vi "Measurer.vi"() -> ()   [LabVIEW 2019]
uses:
  <vilib>/Analysis/baseanly.llb/Mean (DBL).vi
  Components/DeltaRamp_globals.vi
  Components/B_Globals.vi
  Components/Global 2.vi
  Components/ReadLockGlobals.vi
  <vilib>/Analysis/NI_AALBase.lvlib
panel:
  out "T_Set [K]":dbl=1.5
  out "R4":cluster{"X":dbl[], "Y":dbl[]}[](graph)=[{"X"=[1.7047999999999999, 1.7049, 1.7048000000000003, 1.7049, 1.7048000000000003, 1.7049, 1.705, 1.7049, 1.705, 1.7048000000000003, 1.7047000000000003, 1.7045999999999997, 1.7047000000000012, 1.7047999999999999, 1.7045999999999994, 1.7044999999999997, 1.7045999999999997, 1.7044999999999997, 1.7045999999999994, 1.7044999999999997, 1.7046, 1.7044999999999997, 1.7044, 1.7044999999999997, 1.7044, 1.7043, 1.7044, 1.7044999999999997, 1.7044000000000001, 1.7044999999999997, 1.7047000000000003, 1.7045999999999997, 1.7044999999999997, 1.7045999999999997, 1.7046999999999999, 1.7045999999999997, 1.7046999999999999, 1.7048000000000003, 1.7047000000000003, 1.7047999999999994, 1.7049, 1.7047999999999999, 1.7047, 1.7048000000000003, 1.7045999999999997, 1.7047, 1.7048000000000003, 1.7049, 1.7048000000000003], "Y"=[]}] caption="XY Graph"
  out "R [Ohm]":dbl[](array[numeric])=[0.218917653]
  out "Array":T1(array[cluster])=[{"Name"="AEN056B", "Measurment Type"="6221 - Delta", "I Max"=1e-05, "Freq/Delay"=0.002, "Address"="GPIB1::20::INSTR", "Enabled"=FALSE}, {"Name"="CrossJunction_device5", "Measurment Type"="6221 - Delta", "I Max"=1e-05, "Freq/Delay"=0.002, "Address"="GPIB1::22::INSTR", "Enabled"=TRUE}]
  in  "Config":bool
  in  "Graphing":string(combo)="Single"
  out "T 3":cluster{"X":dbl[], "Y":dbl[]}[](graph)=[{"X"=[1.7047999999999999, 1.7049, 1.7048000000000003, 1.7049, 1.7048000000000003, 1.7049, 1.705, 1.7049, 1.705, 1.7048000000000003, 1.7047000000000003, 1.7045999999999997, 1.7047000000000012, 1.7047999999999999, 1.7045999999999994, 1.7044999999999997, 1.7045999999999997, 1.7044999999999997, 1.7045999999999994, 1.7044999999999997, 1.7046, 1.7044999999999997, 1.7044, 1.7044999999999997, 1.7044, 1.7043, 1.7044, 1.7044999999999997, 1.7044000000000001, 1.7044999999999997, 1.7047000000000003, 1.7045999999999997, 1.7044999999999997, 1.7045999999999997, 1.7046999999999999, 1.7045999999999997, 1.7046999999999999, 1.7048000000000003, 1.7047000000000003, 1.7047999999999994, 1.7049, 1.7047999999999999, 1.7047, 1.7048000000000003, 1.7045999999999997, 1.7047, 1.7048000000000003, 1.7049, 1.7048000000000003], "Y"=[]}] caption="XY Graph"
  out "T 2":cluster{"X":dbl[], "Y":dbl[]}[](graph)=[{"X"=[1.7047999999999999, 1.7049, 1.7048000000000003, 1.7049, 1.7048000000000003, 1.7049, 1.705, 1.7049, 1.705, 1.7048000000000003, 1.7047000000000003, 1.7045999999999997, 1.7047000000000012, 1.7047999999999999, 1.7045999999999994, 1.7044999999999997, 1.7045999999999997, 1.7044999999999997, 1.7045999999999994, 1.7044999999999997, 1.7046, 1.7044999999999997, 1.7044, 1.7044999999999997, 1.7044, 1.7043, 1.7044, 1.7044999999999997, 1.7044000000000001, 1.7044999999999997, 1.7047000000000003, 1.7045999999999997, 1.7044999999999997, 1.7045999999999997, 1.7046999999999999, 1.7045999999999997, 1.7046999999999999, 1.7048000000000003, 1.7047000000000003, 1.7047999999999994, 1.7049, 1.7047999999999999, 1.7047, 1.7048000000000003, 1.7045999999999997, 1.7047, 1.7048000000000003, 1.7049, 1.7048000000000003], "Y"=[0.19752289130769227, 0.20950811671428574, 0.1808979382857143, 0.17235231225, 0.17432194683333332, 0.2235183616666667, 0.21412651671428576, 0.20596404375999997, 0.2051939327142857, 0.20028577114285714, 0.19771953790909091, 0.20788647657142859, 0.19616624683333334, 0.1948073679230769, 0.2037684524285714, 0.196056151, 0.196453916, 0.19739343871428575, 0.21256366375, 0.1747552657, 0.15625726666666667, 0.19934746358333333, 0.19194195983333331, 0.19936784685714287, 0.2009971615357143, 0.21071373433333332, 0.20681018633333334, 0.20449920628571427, 0.1755347936, 0.20595055476923077, 0.20658881114285715, 0.21645730942857141, 0.20386924071428572, 0.1994578533809524, 0.20553432800000002, 0.21412651242857142, 0.20646832086666667, 0.2077425187142857, 0.218575714, 0.20290053768181818, 0.17640915285714284, 0.19304051792857146, 0.209842004, 0.2081186685714286, 0.20430601066666668, 0.20083773000000002, 0.19869472714285713, 0.20326516587499996, 0.20483756485714283]}] caption="XY Graph"
  in  "Clear Paths":bool
  out "Remote Inherit Path":path=path "C:/User Data/gy251/20210406 EuS10-Cu (t)-EuS20/Delta_500uA_RH_T=16p00K.txt"
  in  "Remote Directory":path=path "C:/User Data/gy251/20210811 Cross junction for Oded/Device 5_750 nm width/Junction check_7-8-10-11"
  out "Last Saved":path=path "C:/User Data/gy251/20210810 AEN056B/JJ8/CrossJunction_device5_RT_10uA_cool.txt"
  in  "Remote_Save_String [This is the important one!]":string="RT_10uA_warm"
  out "B_set [T]":dbl
  in  "Reading Delay [ms]":i32=20 min=5
  in  "RW Delay":i32=10
  out "Exec Time [ms]":u32=39
  in  "B/T":bool=TRUE
  in  "Smart Avs":bool=TRUE
  in  "Points":dbl=1.0
  out "PpP":dbl=7.0
  in  "Combo Box":string(combo)="Temp"
  in  "Save":bool
  in  "Abort":bool
  out "B [T]":dbl
  in  "Arm":bool
  in  "Measure":bool
  out "T":cluster{"X":dbl[], "Y":dbl[]}[](graph)=[{"X"=[1.7047999999999999, 1.7049, 1.7048000000000003, 1.7049, 1.7048000000000003, 1.7049, 1.705, 1.7049, 1.705, 1.7048000000000003, 1.7047000000000003, 1.7045999999999997, 1.7047000000000012, 1.7047999999999999, 1.7045999999999994, 1.7044999999999997, 1.7045999999999997, 1.7044999999999997, 1.7045999999999994, 1.7044999999999997, 1.7046, 1.7044999999999997, 1.7044, 1.7044999999999997, 1.7044, 1.7043, 1.7044, 1.7044999999999997, 1.7044000000000001, 1.7044999999999997, 1.7047000000000003, 1.7045999999999997, 1.7044999999999997, 1.7045999999999997, 1.7046999999999999, 1.7045999999999997, 1.7046999999999999, 1.7048000000000003, 1.7047000000000003, 1.7047999999999994, 1.7049, 1.7047999999999999, 1.7047, 1.7048000000000003, 1.7045999999999997, 1.7047, 1.7048000000000003, 1.7049, 1.7048000000000003], "Y"=[0.19752289130769227, 0.20950811671428574, 0.1808979382857143, 0.17235231225, 0.17432194683333332, 0.2235183616666667, 0.21412651671428576, 0.20596404375999997, 0.2051939327142857, 0.20028577114285714, 0.19771953790909091, 0.20788647657142859, 0.19616624683333334, 0.1948073679230769, 0.2037684524285714, 0.196056151, 0.196453916, 0.19739343871428575, 0.21256366375, 0.1747552657, 0.15625726666666667, 0.19934746358333333, 0.19194195983333331, 0.19936784685714287, 0.2009971615357143, 0.21071373433333332, 0.20681018633333334, 0.20449920628571427, 0.1755347936, 0.20595055476923077, 0.20658881114285715, 0.21645730942857141, 0.20386924071428572, 0.1994578533809524, 0.20553432800000002, 0.21412651242857142, 0.20646832086666667, 0.2077425187142857, 0.218575714, 0.20290053768181818, 0.17640915285714284, 0.19304051792857146, 0.209842004, 0.2081186685714286, 0.20430601066666668, 0.20083773000000002, 0.19869472714285713, 0.20326516587499996, 0.20483756485714283]}] caption="XY Graph"
  in  "Reset":bool
  out "Spl T [K]":dbl=1.7047
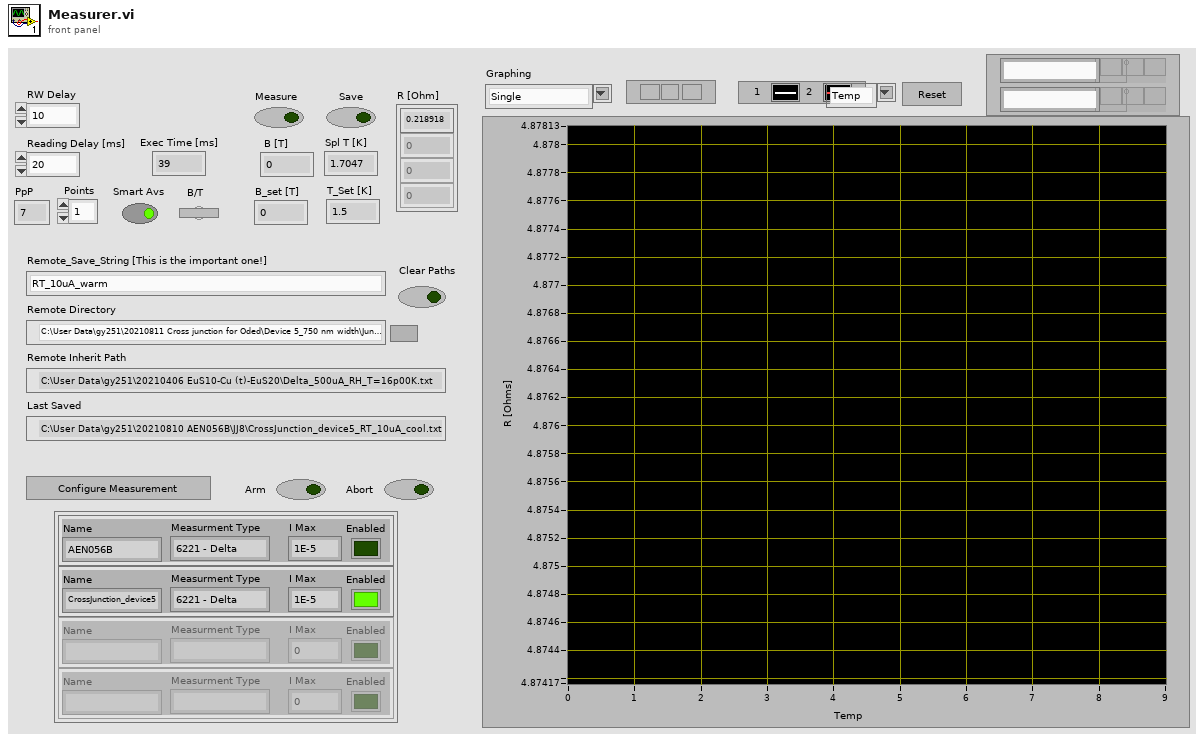
[diagram p1: front panel]
types:
  T1 = cluster{"Name":string, "Measurment Type":string, "I Max":dbl, "Freq/Delay":dbl, "Address":refnum<visa-resource-name>, "Enabled":bool}[]
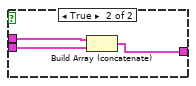
[diagram p4: hidden frame]
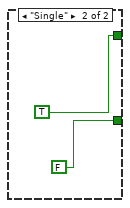
[diagram p5: hidden frame]
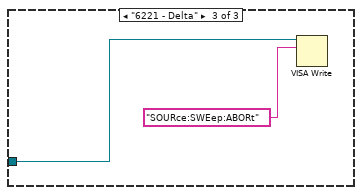
[diagram p8: hidden frame]
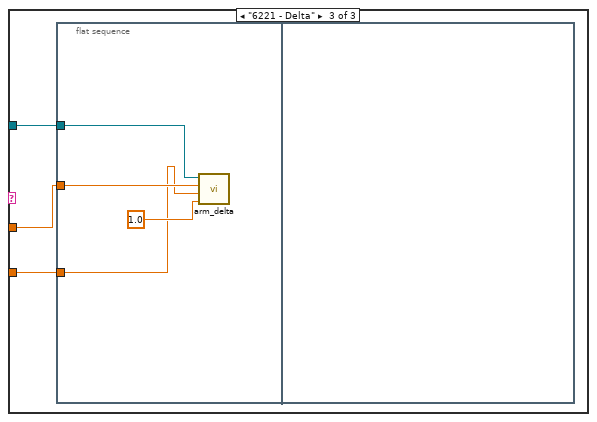
[diagram p12: hidden frame]
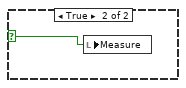
[diagram p13: hidden frame]
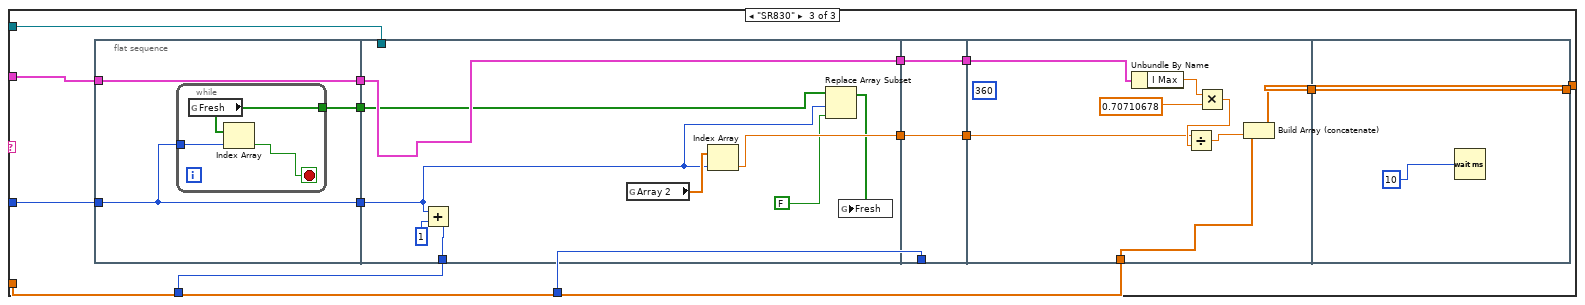
[diagram p18: hidden frame]
diagram:
  # "D2"
  # "D1"
  n1 = while {
    shift-right: [w2] -> _
    shift-left: _ -> [w3]
    stop <- FALSE stop-if-true
    w1 = FALSE
    # "Short T"
    # "Short B"
    n2 = global read "DeltaRamp_globals.vi" "Remote_Measure"() -> (w4:bool)
    n3 = property on="Freq/Delay" class="DigNum (strict)"("Visible"=w1) -> ()  [unwired: 2 in, 2 out]
    n4 = property on="Address" class="VISAName"("Visible"=w1) -> ()  [unwired: 2 in, 2 out]
    n5 = Or(x="Measure", y=w4) -> (x .or. y?=w6:bool)
    n6 = case shown="True" w6 {
      tunnel: w4 -> [_ w78]
      tunnel: w3 -> [w11 w77]
      tunnel: [w10 w77] -> w2
      frame False {
        n7 = case shown="True" "Config" {
          tunnel: w11 -> [w21 _]
          tunnel: [w21 w25] -> w10
          frame False {
          }
          frame True {
            n8 = flat-sequence {
              tunnel: [w27] -> w24
              tunnel: [w27] -> w23
              tunnel: [w26] -> w22
              tunnel: [w26] -> _
              tunnel: [w39] -> w25
              tunnel: w24 -> [_]
              tunnel: w23 -> [w39]
              tunnel: w22 -> [w37]
              frame #0 {
                (unwired) FALSE
                n9 = call "MeasurementConfig.vi"() -> ("Array 2"=w26:T1)  [unwired: 10 in]
                n10 = for {
                  tunnel: w26 -> [w31] mode=indexing
                  shift-right: [w29] -> w27
                  shift-left: T1 [] -> [w30]
                  n11 = Unbundle By Name(w31) -> ("Enabled"=w32:bool)
                  n12 = case shown="False" w32 {
                    tunnel: w31 -> [_ w36]
                    tunnel: w30 -> [w33 w35]
                    tunnel: [w33 w34] -> w29
                    frame False {
                    }
                    frame True {
                      n13 = Build Array (concatenate)(w35, w36) -> (w34:T1)
                    }
                  }
                }
              }
              frame #1 {
                n14 = local write "Config"(FALSE) -> ()
                "Array" <- w37
              }
            }
          }
        }
        n15 = case shown="True" "Arm" {
          tunnel: w10 -> [_ w54]
          frame False {
          }
          frame True {
            n16 = flat-sequence {
              tunnel: w54 -> [w55]
              frame #0 {
                n17 = for {
                  tunnel: w55 -> [w57] mode=indexing
                  n18 = Unbundle By Name(w57) -> ("Measurment Type"=w61:string)
                  n19 = Unbundle By Name(w57) -> ("Enabled"=w56:bool)
                  n20 = Unbundle By Name(w57) -> ("Freq/Delay"=w58:dbl)
                  n21 = Unbundle By Name(w57) -> ("Address"=w60:refnum<visa-resource-name>)
                  n22 = Unbundle By Name(w57) -> ("I Max"=w59:dbl)
                  n23 = case shown="True" w56 {
                    tunnel: w61 -> [_ w65]
                    tunnel: w60 -> [_ w64]
                    tunnel: w59 -> [_ w63]
                    tunnel: w58 -> [_ w62]
                    frame False {
                    }
                    frame True {
                      n24 = case shown="\"6221 - AC\"" w65 {
                        tunnel: w64 -> [_ w66 w71]
                        tunnel: w63 -> [_ w67 w70]
                        tunnel: w62 -> [_ w68 w69]
                        frame "False", Default {
                        }
                        frame "6221 - AC" {
                          n25 = call "arm_sine.vi"("Peak Amp"=w67, "Freq"=w68, "Keithley"=w66) -> ()  [unwired: 9 in]
                        }
                        frame "6221 - Delta" {
                          n26 = flat-sequence {
                            tunnel: w71 -> [w75]
                            tunnel: w70 -> [w73]
                            tunnel: w69 -> [w72]
                            frame #0 {
                              n27 = call "arm_delta.vi"("Compliance [V]"=1.0, "DELAY [sec]"=w72, "I-HIGH [A]"=w73, "Keithley"=w75) -> ()  [unwired: 7 in, 1 out]
                            }
                            frame #1 {
                            }
                          }
                        }
                      }
                    }
                  }
                }
              }
              frame #1 {
                n28 = local write "Arm"(FALSE) -> ()
              }
            }
          }
        }
        n29 = case shown="True" "Abort" {
          tunnel: w10 -> [_ w44]
          frame False {
          }
          frame True {
            n30 = flat-sequence {
              tunnel: w44 -> [w45]
              frame #0 {
                n31 = for {
                  tunnel: w45 -> [w48] mode=indexing
                  n32 = Unbundle By Name(w48) -> ("Measurment Type"=w47:string)
                  n33 = Unbundle By Name(w48) -> ("Address"=w46:refnum<visa-resource-name>)
                  n34 = case shown="\"6221 - AC\"" w47 {
                    tunnel: w46 -> [_ w49 w51]
                    frame "False", Default {
                    }
                    frame "6221 - AC" {
                      n35 = VISA Write(VISA resource name=w49, write buffer="SOUR:WAVE:ABOR") -> ()  [unwired: 1 in, 3 out]
                    }
                    frame "6221 - Delta" {
                      n36 = VISA Write(VISA resource name=w51, write buffer="SOURce:SWEep:ABORt") -> ()  [unwired: 1 in, 3 out]
                    }
                  }
                }
              }
              frame #1 {
                n37 = local write "Abort"(FALSE) -> ()
              }
            }
          }
        }
        n38 = Wait (ms)(milliseconds to wait=500) -> ()  [unwired: 1 out]
        n39 = property on="T" class="XYGraph (strict)"("Active Plot"=0, "Plot.Plot Name"="1", "Active Plot"=1, "Plot.Plot Name"="2") -> ()  [unwired: 2 in, 2 out]
        n40 = local read "Graphing"() -> (w16:string)
        n41 = case shown="\"Dual\", Default" w16 {
          tunnel: [FALSE TRUE] -> w18
          tunnel: [TRUE FALSE] -> w17
          frame "Dual", Default {
          }
          frame "Single" {
          }
        }
        n42 = property on="T 3" class="XYGraph (strict)"("Visible"=w17) -> ()  [unwired: 2 in, 2 out]
        n43 = property on="T 2" class="XYGraph (strict)"("Visible"=w17) -> ()  [unwired: 2 in, 2 out]
        n44 = property on="T" class="XYGraph (strict)"("Visible"=w18) -> ()  [unwired: 2 in, 2 out]
      }
      frame True {
        # "Ramp=False?"
        n45 = case shown="False" w78 {
          selector: w78 -> [_ w79]
          frame False {
          }
          frame True {
            n46 = local write "Measure"(w79) -> ()
          }
        }
        n47 = while {
          shift-right: [w137] -> _
          shift-left: _ -> [w141]
          shift-right: [w146] -> _
          shift-left: _ -> [w152]
          shift-right: [w136] -> _
          shift-left: _ -> [w144]
          shift-right: [w147] -> _
          shift-left: _ -> [w155]
          shift-right: [w160] -> _
          shift-left: _ -> [w161]
          shift-right: [w163] -> _
          shift-left: _ -> [w164]
          shift-right: [w123] -> _
          shift-left: _ -> [w127]
          shift-right: [w115] -> _
          shift-left: _ -> [w119]
          shift-right: [w113] -> _
          shift-left: _ -> [w111]
          tunnel: w77 -> [w94]
          shift-right: [w80] -> _
          shift-left: _ -> [w87]
          stop <- w129 stop-if-true
          # "T_Set"
          # "R2"
          n48 = global write "DeltaRamp_globals.vi" "Remote_Measure"(FALSE) -> ()
          n49 = flat-sequence {
            tunnel: w164 -> [w177]
            tunnel: [w175] -> w163
            tunnel: w155 -> [w174]
            tunnel: [w174] -> w154
            tunnel: w152 -> [w173]
            tunnel: [w173] -> w150
            tunnel: [w172] -> w145
            tunnel: w144 -> [w172]
            tunnel: [w171] -> w142
            tunnel: w141 -> [w171]
            tunnel: [w170] -> w128
            tunnel: w127 -> [w170]
            tunnel: [w169] -> w120
            tunnel: w119 -> [w169]
            tunnel: [w168] -> w112
            tunnel: w111 -> [w168]
            tunnel: w94 -> [w167]
            tunnel: [w167] -> w92
            tunnel: w87 -> [w166]
            tunnel: [w166] -> w85
            tunnel: w154 -> [w189]
            tunnel: [w189] -> w108
            tunnel: [w188] -> w106
            tunnel: w150 -> [w188]
            tunnel: w145 -> [w187]
            tunnel: [w187] -> w104
            tunnel: w142 -> [w186]
            tunnel: [w186] -> w102
            tunnel: w128 -> [w185]
            tunnel: [w185] -> w100
            tunnel: w120 -> [w184]
            tunnel: [w184] -> w98
            tunnel: w112 -> [w183]
            tunnel: [w183] -> w96
            tunnel: [w182] -> w93
            tunnel: w92 -> [w182]
            tunnel: [w178] -> w86
            tunnel: w85 -> [w178]
            tunnel: w108 -> [w202]
            tunnel: [w202] -> w107
            tunnel: w106 -> [w201]
            tunnel: [w201] -> w105
            tunnel: w104 -> [w200]
            tunnel: [w200] -> w103
            tunnel: w102 -> [w199]
            tunnel: [w199] -> w101
            tunnel: w100 -> [w198]
            tunnel: [w198] -> w99
            tunnel: w98 -> [w197]
            tunnel: [w197] -> w97
            tunnel: w96 -> [w196]
            tunnel: [w196] -> w95
            tunnel: w93 -> [w194]
            tunnel: [w194] -> w90
            tunnel: w86 -> [w193]
            tunnel: [w193] -> w83
            tunnel: [w222] -> w159
            tunnel: [w221] -> w157
            tunnel: w107 -> [w220]
            tunnel: [w220] -> w153
            tunnel: [w219] -> w151
            tunnel: w105 -> [w219]
            tunnel: [w218] -> w143
            tunnel: w103 -> [w218]
            tunnel: [w217] -> w140
            tunnel: w101 -> [w217]
            tunnel: [w216] -> w126
            tunnel: w99 -> [w216]
            tunnel: [w215] -> w122
            tunnel: w97 -> [w214]
            tunnel: [w214] -> w117
            tunnel: [w213] -> w110
            tunnel: w95 -> [w213]
            tunnel: [w212] -> w91
            tunnel: w90 -> [w212]
            tunnel: [w211] -> w84
            tunnel: w83 -> [w211]
            tunnel: [w238] -> w162
            tunnel: w161 -> [w238]
            tunnel: w159 -> [w237]
            tunnel: [w237] -> w158
            tunnel: w157 -> [w236]
            tunnel: [w236] -> w156
            tunnel: w153 -> [w235]
            tunnel: w151 -> [w234]
            tunnel: [w235] -> w149
            tunnel: [w234] -> w148
            tunnel: w143 -> [w233]
            tunnel: w140 -> [w232]
            tunnel: [w233] -> w139
            tunnel: [w232] -> w138
            tunnel: ["Points"] -> w135
            tunnel: w126 -> [w230]
            tunnel: [w230] -> w125
            tunnel: w122 -> [w229]
            tunnel: [w229] -> w121
            tunnel: [w228] -> w118
            tunnel: w117 -> [w228]
            tunnel: w110 -> [w227]
            tunnel: [w227] -> w109
            tunnel: w91 -> [w226]
            tunnel: [w226] -> w89
            tunnel: [w224] -> w88
            tunnel: w84 -> [w223]
            tunnel: [w223] -> w82
            tunnel: w162 -> [w409]
            tunnel: w158 -> [w404]
            tunnel: w156 -> [w400]
            tunnel: w149 -> [w405]
            tunnel: w148 -> [w403]
            tunnel: w139 -> [w392]
            tunnel: w138 -> [w391]
            tunnel: w135 -> [w396]
            tunnel: [w397] -> w134
            tunnel: [w402] -> w133
            tunnel: [w401] -> w132
            tunnel: [w399] -> w131
            tunnel: [w398] -> w130
            tunnel: w125 -> [w393]
            tunnel: [w395] -> w124
            tunnel: w121 -> [w390]
            tunnel: w118 -> [w389]
            tunnel: [w387] -> w116
            tunnel: [w357] -> w114
            tunnel: w109 -> [w385]
            tunnel: w89 -> [w375]
            tunnel: w88 -> [w374]
            tunnel: w82 -> [w338]
            tunnel: [w339] -> w81
            tunnel: [w665] -> w136
            tunnel: [w666] -> w137
            tunnel: [w667] -> w146
            tunnel: [w668] -> w147
            tunnel: [w669] -> w160
            tunnel: w134 -> [w669]
            tunnel: w133 -> [w668]
            tunnel: w132 -> [w667]
            tunnel: w131 -> [w666]
            tunnel: w130 -> [w665]
            tunnel: w124 -> [w663]
            tunnel: [w663] -> w123
            tunnel: [w662] -> w115
            tunnel: w116 -> [w662]
            tunnel: w114 -> [w661]
            tunnel: [w661] -> w113
            tunnel: [w660] -> w80
            tunnel: w81 -> [w660]
            frame #0 {
              n50 = Tick Count (ms)() -> (millisecond timer value=w175:u32)
              n51 = Subtract(x=w175, y=w177) -> (x-y=→"Exec Time [ms]":u32)
            }
            frame #1 {
              n52 = global read "DeltaRamp_globals.vi" "Remote_Save_String"() -> (w180:string)
              n53 = Not Equal?(x=w180, y="") -> (x != y?=w179:bool)
              n54 = case shown="True" w179 {
                frame False {
                }
                frame True {
                  n55 = global read "DeltaRamp_globals.vi" "Remote_Save_Directory"() -> (w191:path)
                  n56 = global read "DeltaRamp_globals.vi" "Remote_Save_String"() -> (w192:string)
                  n57 = global read "DeltaRamp_globals.vi" "Remote_Ramp_Path"() -> (w190:path)
                  n58 = local write "Remote_Save_String [This is the important one!]"(w192) -> ()
                  n59 = local write "Remote Directory"(w191) -> ()
                  n60 = local write "Remote Inherit Path"(w190) -> ()
                }
              }
            }
            frame #2 {
              n61 = case shown="True" "Clear Paths" {
                frame False {
                }
                frame True {
                  n62 = flat-sequence {
                    tunnel: [w206] -> w204
                    tunnel: [w205] -> w203
                    tunnel: w204 -> [w208]
                    tunnel: w203 -> [w207]
                    frame #0 {
                      w205 = path ""
                      w206 = ""
                      n63 = global write "DeltaRamp_globals.vi" "Remote_Save_Directory"(w205) -> ()
                      n64 = global write "DeltaRamp_globals.vi" "Remote_Save_String"(w206) -> ()
                      n65 = global write "DeltaRamp_globals.vi" "Remote_Ramp_Path"(w205) -> ()
                    }
                    frame #1 {
                      n66 = local write "Remote_Save_String [This is the important one!]"(w208) -> ()
                      n67 = local write "Remote Directory"(w207) -> ()
                    }
                    frame #2 {
                      n68 = local write "Clear Paths"(FALSE) -> ()
                    }
                  }
                }
              }
            }
            frame #3 {
              n69 = global read "Global 2.vi" "G_Sample_Set"() -> (→"T_Set [K]":dbl)
              n70 = global read "Global 2.vi" "SampleTemp"() -> (w221:dbl)
              "Spl T [K]" <- w221
              n71 = global read "B_Globals.vi" "G_B_set[T]"() -> (w215:dbl)
              "B_set [T]" <- w215
              n72 = global read "B_Globals.vi" "B [T]"() -> (w222:dbl)
              "B [T]" <- w222
            }
            frame #4 {
              # "R2"
              # "Bset"
              # "Points"
              # "Short R"
              # "New T"
              # "New B"
              # "Short T"
              # "Short B"
              # "New R"
              n73 = flat-sequence {
                tunnel: "RW Delay" -> [w243]
                tunnel: w226 -> [w242]
                tunnel: [w240] -> w224
                frame #0 {
                  n74 = for {
                    tunnel: w243 -> [w251]
                    tunnel: w242 -> [w247] mode=indexing
                    shift-right: [w248] -> w240
                    shift-left: dbl[] [] -> [w249]
                    shift-right: [w244] -> _
                    shift-left: 0 -> [w245]
                    # "SR830 Count"
                    n75 = Unbundle By Name(w247) -> ("Measurment Type"=w246:string)
                    n76 = Unbundle By Name(w247) -> ("Enabled"=w250:bool)
                    n77 = case shown="True" w250 {
                      tunnel: [w253 w261] -> w248
                      tunnel: w251 -> [_ w260]
                      tunnel: w247 -> [_ w257]
                      tunnel: w249 -> [w253 w259]
                      tunnel: w246 -> [_ w258]
                      tunnel: w245 -> [w252 w255]
                      tunnel: [w252 w254] -> w244
                      frame False {
                      }
                      frame True {
                        n78 = Unbundle By Name(w257) -> ("Address"=w256:refnum<visa-resource-name>)
                        n79 = case shown="\"6221 - Delta\"" w258 {
                          tunnel: [w263 w265 w305] -> w261
                          tunnel: w260 -> [_ w267 w304]
                          tunnel: w257 -> [_ w268 w303]
                          tunnel: w259 -> [w263 w266 w302]
                          tunnel: w256 -> [_ _ w301]
                          tunnel: w255 -> [w262 w264 w300]
                          tunnel: [w262 w264 w299] -> w254
                          frame "False", Default {
                          }
                          frame "6221 - Delta" {
                            n80 = flat-sequence {
                              tunnel: [w280] -> w275
                              tunnel: [w276] -> w274
                              tunnel: [w277] -> w273
                              tunnel: w268 -> [w276]
                              tunnel: [w284] -> w272
                              tunnel: w275 -> [w284]
                              tunnel: w267 -> [w283]
                              tunnel: w274 -> [w282]
                              tunnel: [w282] -> w271
                              tunnel: [w281] -> w270
                              tunnel: w273 -> [w281]
                              tunnel: w272 -> [w291]
                              tunnel: [w290] -> w269
                              tunnel: w266 -> [w286]
                              tunnel: w271 -> [_]
                              tunnel: w270 -> [_]
                              tunnel: [w293] -> w265
                              tunnel: w269 -> [w293]
                              frame #0 {
                                n81 = Unbundle By Name(w276) -> ("Address"=w278:refnum<visa-resource-name>)
                                n82 = Unbundle By Name(w276) -> ("Measurment Type"=w277:string)
                                n83 = VISA Write(VISA resource name=w278, write buffer="SENS:DATA:FRESh?") -> (VISA resource name out=w280:refnum<visa-resource-name>)  [unwired: 1 in, 2 out]
                              }
                              frame #1 {
                                n84 = Wait (ms)(milliseconds to wait=w283) -> ()  [unwired: 1 out]
                              }
                              frame #2 {
                                n85 = VISA Read(VISA resource name=w291, byte count=u32 360) -> (read buffer=w288:string)  [unwired: 1 in, 3 out]
                                n86 = Search/Split String(string=w288, search string/char (-)=",") -> (substring before match=w287:string)  [unwired: 1 in, 2 out]
                                n87 = Fract/Exp String To Number(string=w287) -> (number=w285:dbl)  [unwired: 1 in, 3 out]
                                n88 = Build Array (concatenate)(w286, w285) -> (w290:dbl[])
                              }
                              frame #3 {
                              }
                            }
                          }
                          frame "SR830" {
                            n89 = flat-sequence {
                              tunnel: w300 -> [w310]
                              tunnel: w303 -> [w311]
                              tunnel: [w311] -> w296
                              tunnel: [w310] -> w295
                              tunnel: [w309] -> w294
                              tunnel: [w323] -> w308
                              tunnel: w301 -> [_]
                              tunnel: [w321] -> w299
                              tunnel: [w319] -> w297
                              tunnel: w296 -> [w323]
                              tunnel: w295 -> [w318]
                              tunnel: w294 -> [w315]
                              tunnel: w304 -> [_]
                              tunnel: w308 -> [w325]
                              tunnel: [w325] -> w307
                              tunnel: [w324] -> w298
                              tunnel: w297 -> [w324]
                              tunnel: [w333] -> w306
                              tunnel: w302 -> [w332]
                              tunnel: w307 -> [w331]
                              tunnel: w298 -> [w326]
                              tunnel: [w335] -> w305
                              tunnel: w306 -> [w335]
                              frame #0 {
                                n90 = while {
                                tunnel: w310 -> [w314]
                                tunnel: [w312] -> w309
                                stop <- w313 stop-if-true
                                n91 = global read "ReadLockGlobals.vi" "Fresh"() -> (w312:bool[])
                                n92 = Index Array(array=w312, index=w314) -> (element=w313:bool)
                                }
                              }
                              frame #1 {
                                n93 = Add(x=w318, y=1) -> (x+y=w321:i32)
                                n94 = global read "ReadLockGlobals.vi" "Array 2"() -> (w320:dbl[])
                                n95 = Index Array(array=w320, index=w318) -> (element=w319:dbl)
                                n96 = Replace Array Subset(array=w315, new element=FALSE, index=w318) -> (w316:bool[])
                                n97 = global write "ReadLockGlobals.vi" "Fresh"(w316) -> ()
                              }
                              frame #2 {
                              }
                              frame #3 {
                                (unwired) u32 360 ("byte count")
                                n98 = Unbundle By Name(w331) -> ("I Max"=w329:dbl)
                                n99 = Multiply(x=w329, y=0.70710678) -> (x*y=w327:dbl)
                                n100 = Divide(x=w326, y=w327) -> (x/y=w330:dbl)
                                n101 = Build Array (concatenate)(w332, w330) -> (w333:dbl[])
                              }
                              frame #4 {
                                n102 = Wait (ms)(milliseconds to wait=10) -> ()  [unwired: 1 out]
                              }
                            }
                          }
                        }
                      }
                    }
                  }
                }
              }
            }
            frame #5 {
              (unwired) 1
              (unwired) "1"
              (unwired) 1
              (unwired) 0
              # "PpP"
              n103 = global read "DeltaRamp_globals.vi" "Remote_Ramp_Save"() -> (w418:bool)
              n104 = Delete From Array(array=w403) -> (deleted portion=w407:dbl)  [unwired: 2 in, 1 out]
              n105 = Delete From Array(array=w405) -> (deleted portion=w406:dbl)  [unwired: 2 in, 1 out]
              n106 = Or(x="Save", y=w418) -> (x .or. y?=w413:bool)
              n107 = case shown="True" w413 {
                tunnel: w418 -> [_ w538]
                tunnel: w409 -> [_ w537]
                tunnel: w393 -> [_ w534]
                tunnel: w392 -> [_ w536]
                tunnel: w391 -> [_ w535]
                tunnel: w385 -> [_ w533]
                tunnel: "Save" -> [_ w532]
                tunnel: w375 -> [w527 w530]
                tunnel: [w527 w529] -> w353
                tunnel: w338 -> [_ w528]
                frame False {
                }
                frame True {
                  n108 = flat-sequence {
                    tunnel: w538 -> [w555]
                    tunnel: w537 -> [w550]
                    tunnel: w536 -> [w552]
                    tunnel: w535 -> [w551]
                    tunnel: w534 -> [w549]
                    tunnel: w533 -> [w553]
                    tunnel: w530 -> [w548]
                    tunnel: [w548] -> w529
                    tunnel: w528 -> [w539]
                    tunnel: w532 -> [w637]
                    tunnel: [w638] -> w531
                    tunnel: w531 -> [_]
                    frame #0 {
                      (unwired) path ""
                      (unwired) ""
                      # "BSet"
                      # "PpP"
                      # "D1"
                      # "L1"
                      # "T"
                      # "B"
                      n109 = local read "Remote_Save_String [This is the important one!]"() -> (w541:string)
                      n110 = local read "Remote Directory"() -> (w542:path)
                      n111 = Not Equal?(x=w541, y="") -> (x != y?=w546:bool)
                      n112 = Not Equal?(x=w542, y=path "") -> (x != y?=w545:bool)
                      n113 = Or(x=w546, y=w545) -> (x .or. y?=w543:bool)
                      n114 = Concatenate Strings("2", "_", w541) -> (w557:string)
                      n115 = Build Path(base path=w542, name or relative path=w557) -> ()  [unwired: 1 out]
                      n116 = for {
                        tunnel: w542 -> [w584]
                        tunnel: w555 -> [w583]
                        tunnel: w543 -> [w564]
                        tunnel: w548 -> [w566] mode=indexing
                        tunnel: w553 -> [w572]
                        tunnel: w552 -> [w581]
                        tunnel: w551 -> [w579]
                        tunnel: w550 -> [w576]
                        tunnel: w549 -> [w575]
                        tunnel: w541 -> [w563]
                        tunnel: 0 -> [w560]
                        tunnel: w539 -> [w559]
                        i -> [w571]
                        n117 = Unbundle By Name(w566) -> ("Enabled"=w561:bool)
                        n118 = Unbundle By Name(w566) -> ("Name"=w567:string)
                        n119 = Index Array(array=w572, index (col)=w571) -> (element=w570:dbl[])  [unwired: 1 in]
                        n120 = case shown="True" w561 {
                          tunnel: w560 -> [_ w587]
                          frame False {
                          }
                          frame True {
                            n121 = Add(x=w587, y=0) -> ()  [unwired: 1 out]
                          }
                        }
                        n122 = Unbundle By Name(w566) -> ("Measurment Type"=w565:string)
                        n123 = call "Convert to Dynamic Data3"("Array"=w581) -> ("Dynamic Data Type"=w580:dynamicdata)  [unwired: 3 in]
                        n124 = call "Convert to Dynamic Data17"("Array"=w579) -> ("Dynamic Data Type"=w578:dynamicdata)  [unwired: 3 in]
                        n125 = call "Convert to Dynamic Data5"("Array"=w570) -> ("Dynamic Data Type"=w577:dynamicdata)  [unwired: 3 in]
                        n126 = call "Convert to Dynamic Data"("Array"=w576) -> ("Dynamic Data Type"=w574:dynamicdata)  [unwired: 3 in]
                        n127 = call "Convert to Dynamic Data8"("Array"=w559) -> ("Dynamic Data Type"=w558:dynamicdata)  [unwired: 3 in]
                        n128 = Concatenate Strings(w567, "_", w563, ".txt") -> (w569:string)
                        n129 = Build Path(base path=w584, name or relative path=w569) -> (appended path=w585:path)
                        n130 = call "Convert to Dynamic Data4"("Array"=w575) -> ("Dynamic Data Type"=w573:dynamicdata)  [unwired: 3 in]
                        n131 = Merge Signals(w580, w578, w577, w574, w573, w558) -> (w582:dynamicdata)
                        n132 = case shown="\"6221 - Delta\"" w565 {
                          tunnel: w585 -> [_ w592 w617]
                          tunnel: w583 -> [_ w591 w616]
                          tunnel: w564 -> [_ w590 w615]
                          tunnel: w561 -> [_ w589 w614]
                          tunnel: w582 -> [_ w588 w613]
                          frame "False", Default {
                          }
                          frame "6221 - Delta" {
                            n133 = case shown="True" w589 {
                              tunnel: w588 -> [_ w596]
                              tunnel: w590 -> [_ w595]
                              tunnel: w591 -> [_ w594]
                              tunnel: w592 -> [_ w593]
                              frame False {
                              }
                              frame True {
                                n134 = flat-sequence {
                                tunnel: w596 -> [w601]
                                tunnel: w595 -> [w600]
                                tunnel: [w599] -> w597
                                tunnel: w593 -> [w598]
                                tunnel: w597 -> [w608]
                                tunnel: w594 -> [w610]
                                frame #0 {
                                n135 = case shown="True" w600 {
                                tunnel: w601 -> [w603 w607]
                                tunnel: [w602 w606] -> w599
                                tunnel: w598 -> [_ w605]
                                frame False {
                                n136 = call "Write To Measurement File"("Signals"=w603, "Reset"=TRUE) -> ("Filename Out"=w602:path)  [unwired: 15 in, 2 out]
                                }
                                frame True {
                                n137 = call "Write To Measurement File2"("Signals"=w607, "Filename"=w605) -> ("Filename Out"=w606:path)  [unwired: 15 in, 2 out]
                                }
                                }
                                }
                                frame #1 {
                                n138 = call <vilib>:"Is Path and Not Empty.vi"("path"=w608) -> ("Is Path and Not Empty?"=w609:bool)  [unwired: 4 in]
                                n139 = local write "Last Saved"(w608) -> ()
                                n140 = case shown="True" w610 {
                                tunnel: w609 -> [_ w611]
                                frame False {
                                }
                                frame True {
                                n141 = local write "Reset"(w611) -> ()
                                }
                                }
                                }
                                frame #2 {
                                n142 = Wait (ms)(milliseconds to wait=100) -> ()  [unwired: 1 out]
                                }
                                }
                              }
                            }
                          }
                          frame "SR830" {
                            n143 = case shown="True" w614 {
                              tunnel: w613 -> [_ w621]
                              tunnel: w615 -> [_ w620]
                              tunnel: w616 -> [_ w619]
                              tunnel: w617 -> [_ w618]
                              frame False {
                              }
                              frame True {
                                n144 = flat-sequence {
                                tunnel: w621 -> [w626]
                                tunnel: w620 -> [w625]
                                tunnel: [w624] -> w622
                                tunnel: w618 -> [w623]
                                tunnel: w622 -> [w633]
                                tunnel: w619 -> [w635]
                                frame #0 {
                                n145 = case shown="False" w625 {
                                tunnel: w626 -> [w628 w632]
                                tunnel: [w627 w631] -> w624
                                tunnel: w623 -> [_ w630]
                                frame False {
                                n146 = call "Write To Measurement File4"("Signals"=w628, "Reset"=TRUE) -> ("Filename Out"=w627:path)  [unwired: 15 in, 2 out]
                                }
                                frame True {
                                n147 = call "Write To Measurement File3"("Signals"=w632, "Filename"=w630) -> ("Filename Out"=w631:path)  [unwired: 15 in, 2 out]
                                }
                                }
                                }
                                frame #1 {
                                (unwired) ""
                                n148 = call <vilib>:"Is Path and Not Empty.vi"("path"=w633) -> ("Is Path and Not Empty?"=w634:bool)  [unwired: 4 in]
                                n149 = local write "Last Saved"(w633) -> ()
                                n150 = case shown="True" w635 {
                                tunnel: w634 -> [_ w636]
                                frame False {
                                }
                                frame True {
                                n151 = local write "Reset"(w636) -> ()
                                }
                                }
                                }
                                frame #2 {
                                }
                                }
                              }
                            }
                          }
                        }
                      }
                    }
                    frame #1 {
                      n152 = global write "DeltaRamp_globals.vi" "Remote_Skip"(w637) -> ()
                    }
                    frame #2 {
                      w638 = FALSE
                      n153 = global write "DeltaRamp_globals.vi" "Remote_Ramp_Save"(w638) -> ()
                      n154 = local write "Save"(w638) -> ()
                    }
                    frame #3 {
                    }
                  }
                }
              }
              n155 = Array Size(array=w403) -> (size(s)=w423:i32)
              n156 = Not Equal?(x=w407, y=w400) -> (x != y?=w424:bool)
              n157 = Not Equal?(x=w404, y=w406) -> (x != y?=w427:bool)
              n158 = Greater?(x=w423, y=1) -> (0:w426:bool)
              n159 = And(x=w426, y=w427) -> (x .and. y?=w428:bool)
              n160 = And(x=w426, y=w424) -> (x .and. y?=w429:bool)
              n161 = case shown="True" "B/T" {
                tunnel: w428 -> [w462 _]
                tunnel: w429 -> [_ w463]
                tunnel: [w462 w463] -> w430
                frame False {
                  # "B"
                }
                frame True {
                  # "T"
                }
              }
              n162 = Not(x="Smart Avs") -> (.not. x?=w420:bool)
              n163 = Or(x=w420, y=w430) -> (x .or. y?=w421:bool)
              n164 = case shown="False" w421 {
                tunnel: [w472 w499] -> w432
                tunnel: [w471 w489] -> w431
                tunnel: [w469 w497] -> w411
                tunnel: [w470 w495] -> w412
                tunnel: [w473 w494] -> w408
                tunnel: w409 -> [w473 w493]
                tunnel: w405 -> [w472 w486]
                tunnel: w403 -> [w471 w490]
                tunnel: w392 -> [w469 w488]
                tunnel: w391 -> [w470 w487]
                tunnel: w396 -> [_ w485]
                tunnel: w393 -> [w468 w484]
                tunnel: [w468 w483] -> w394
                tunnel: w390 -> [_ w482]
                tunnel: w389 -> [w467 w481]
                tunnel: [w467 w480] -> w388
                tunnel: [w466 w479] -> w386
                tunnel: w385 -> [w466 w478]
                tunnel: w338 -> [w465 w476]
                tunnel: [w465 w474] -> w340
                frame False {
                }
                frame True {
                  # "R"
                  # "T"
                  # "B"
                  n165 = flat-sequence {
                    tunnel: [w510] -> w498
                    tunnel: [w511] -> w496
                    tunnel: w486 -> [w509]
                    tunnel: w490 -> [w508]
                    tunnel: w481 -> [w502]
                    tunnel: [w500] -> w477
                    tunnel: [dbl[] []] -> w489
                    tunnel: [dbl[] []] -> w499
                    tunnel: [dbl[][] []] -> w480
                    frame #0 {
                      n166 = Index Array(array=w502, index (col)=1) -> ()  [unwired: 1 in, 1 out]
                      n167 = call-poly <vilib>:"Mean.vi"("X"=w508) -> ("mean"=w511:dbl)  [unwired: 1 out]
                      n168 = Index Array(array=w502, index (col)=0) -> ()  [unwired: 1 in, 1 out]
                      n169 = call-poly <vilib>:"Mean.vi"("X"=w509) -> ("mean"=w510:dbl)  [unwired: 1 out]
                      n170 = Array Size(array=w502) -> (size(s)=w505:i32[])
                      n171 = Index Array(array=w505, index=1) -> (element=w503:i32)
                      n172 = for {
                        N: w503 -> [_]
                        shift-right: [w513] -> w500
                        shift-left: dbl[] [] -> [w514]
                        tunnel: w502 -> [w517]
                        i -> [w516]
                        n173 = Index Array(array=w517, index (col)=w516) -> (element=w515:dbl[])  [unwired: 1 in]
                        n174 = call-poly <vilib>:"Mean.vi"("X"=w515) -> ("mean"=w512:dbl)  [unwired: 1 out]
                        n175 = Build Array (concatenate)(w514, w512) -> (w513:dbl[])
                      }
                    }
                    frame #1 {
                    }
                  }
                  n176 = Array Size(array=w486) -> (size(s)=w492:i32)
                  n177 = Multiply(x=w492, y=w485) -> (x*y=w491:dbl)
                  "PpP" <- w491
                  n178 = Build Array (concatenate)(w487, w496) -> (w495:dbl[])
                  n179 = Build Array (concatenate)(w488, w498) -> (w497:dbl[])
                  n180 = Build Array (concatenate)(w493, w491) -> (w494:dbl[])
                  n181 = Build Array (concatenate)(w478, w477) -> (w479:dbl[][])
                  n182 = Build Array (concatenate)(w484, w482) -> (w483:dbl[])
                  n183 = global read "Global 2.vi" "G_Sample_Set"() -> (w475:dbl)
                  n184 = Build Array (concatenate)(w476, w475) -> (w474:dbl[])
                }
              }
              n185 = global read "DeltaRamp_globals.vi" "Remote_Reset"() -> (w414:bool)
              n186 = Or(x="Reset", y=w414) -> (x .or. y?=w416:bool)
              n187 = Build Array (concatenate)(w431, w400) -> (w401:dbl[])
              n188 = case shown="False" w416 {
                tunnel: w411 -> [w644 w653]
                tunnel: [w644 w652] -> w398
                tunnel: w412 -> [w643 w651]
                tunnel: [w643 w650] -> w399
                tunnel: [w642 w648] -> w397
                tunnel: w408 -> [w642 _]
                tunnel: [w641 w647] -> w395
                tunnel: w394 -> [w641 _]
                tunnel: w386 -> [w640 _]
                tunnel: [w640 w646] -> w357
                tunnel: w340 -> [w639 _]
                tunnel: [w639 w645] -> w339
                frame False {
                }
                frame True {
                  w649 = FALSE
                  n189 = flat-sequence {
                    tunnel: w653 -> [_]
                    tunnel: w651 -> [_]
                    tunnel: [dbl[] []] -> w650
                    tunnel: [dbl[] []] -> w652
                    tunnel: [dbl[] [] ("Numeric")] -> w648
                    tunnel: [dbl[] [] ("Numeric")] -> w647
                    tunnel: [dbl[][] [] ("Numeric")] -> w646
                    tunnel: [dbl[] [] ("Numeric")] -> w645
                    frame #0 {
                    }
                  }
                  n190 = global write "DeltaRamp_globals.vi" "Remote_Reset"(w649) -> ()
                  n191 = local write "Reset"(w649) -> ()
                }
              }
              n192 = global read "DeltaRamp_globals.vi" "Remote_Req_Stop"() -> (w417:bool)
              n193 = Build Array (concatenate)(w432, w404) -> (w402:dbl[])
              n194 = Build Array (concatenate)(w388, w374) -> (w387:dbl[][])
              n195 = Array Size(array=w357) -> (size(s)=w369:i32[])
              n196 = case shown="\"Temp\"" "Combo Box" {
                tunnel: w399 -> [_ w525]
                tunnel: w398 -> [w523 _]
                tunnel: [w523 w525] -> w381
                tunnel: ["Field" "Temp"] -> w337
                tunnel: [w523 w525] -> w366
                tunnel: ["T" "K"] -> w336
                frame "Field", Default {
                }
                frame "Temp" {
                }
              }
              n197 = Index Array(array=w369, index=1) -> (element=w367:i32)
              n198 = for {
                tunnel: w353 -> [w435] mode=indexing
                shift-right: [w433] -> w349
                shift-left: string[] [] -> [w434]
                n199 = Unbundle By Name(w435) -> ("Enabled"=w436:bool)
                n200 = case shown="True" w436 {
                  tunnel: w435 -> [_ w442]
                  tunnel: w434 -> [w437 w440]
                  tunnel: [w437 w438] -> w433
                  frame False {
                  }
                  frame True {
                    n201 = Unbundle By Name(w442) -> ("Measurment Type"=w441:string)
                    n202 = Unbundle By Name(w442) -> ("Name"=w439:string)
                    n203 = case shown="\"6221 - Delta\"" w441 {
                      tunnel: w440 -> [w443 w445 w449]
                      tunnel: w439 -> [_ w446 w448]
                      tunnel: [w443 w444 w447] -> w438
                      frame "False", Default {
                      }
                      frame "SR830" {
                        n204 = Build Array (concatenate)(w445, w446) -> (w444:string[])
                      }
                      frame "6221 - Delta" {
                        n205 = Build Array (concatenate)(w449, w448) -> (w447:string[])
                      }
                    }
                  }
                }
              }
              n206 = case shown="False" w417 {
                frame False {
                }
                frame True {
                  w464 = FALSE
                  n207 = global write "DeltaRamp_globals.vi" "Remote_Req_Stop"(w464) -> ()
                  n208 = local write "Measure"(w464) -> ()
                }
              }
              n209 = Index Array(array=w357, index (col)=0) -> (element=w373:dbl[])  [unwired: 1 in]
              n210 = Index Array(array=w357, index (col)=2) -> (element=w356:dbl[])  [unwired: 1 in]
              n211 = Index Array(array=w357, index (col)=1) -> (element=w370:dbl[])  [unwired: 1 in]
              n212 = call "Convert to Dynamic Data15"("Array"=w381) -> ("Dynamic Data Type"=w359:dynamicdata)  [unwired: 3 in]
              n213 = call "Convert to Dynamic Data16"("Array"=w370) -> ("Dynamic Data Type"=w380:dynamicdata)  [unwired: 3 in]
              n214 = for {
                N: w367 -> [_]
                shift-right: [w454] -> w363
                shift-left: dbl[][] [] -> [w455]
                shift-right: [w456] -> w365
                shift-left: dbl[][] [] -> [w457]
                tunnel: w366 -> [w453]
                tunnel: w357 -> [w452]
                i -> [w451]
                n215 = Index Array(array=w452, index (col)=w451) -> (element=w450:dbl[])  [unwired: 1 in]
                n216 = Build Array (concatenate)(w457, w450) -> (w456:dbl[][])
                n217 = Build Array (concatenate)(w455, w453) -> (w454:dbl[][])
              }
              n218 = call "Convert to Dynamic Data14"("Array"=w381) -> ("Dynamic Data Type"=w382:dynamicdata)  [unwired: 3 in]
              n219 = call "Convert to Dynamic Data13"("Array"=w373) -> ("Dynamic Data Type"=w383:dynamicdata)  [unwired: 3 in]
              n220 = call "Build XY Graph3"("Y Input"=w380, "X Input"=w359) -> ("XY Graph"=→"T 3":cluster{"X":dbl[], "Y":dbl[]}[])  [unwired: 8 in, 1 out]
              n221 = case shown="\"Single\"" "Graphing" {
                tunnel: [TRUE FALSE] -> w341
                tunnel: [FALSE TRUE] -> w376
                frame "Multi", Default {
                }
                frame "Single" {
                }
              }
              n222 = call "Build XY Graph"("Y Input"=w383, "X Input"=w382) -> ("XY Graph"=→"T 2":cluster{"X":dbl[], "Y":dbl[]}[])  [unwired: 8 in, 1 out]
              n223 = call "Convert to Dynamic Data7"("Array"=w356) -> ("Dynamic Data Type"=w355:dynamicdata)  [unwired: 3 in]
              n224 = call "Build XY Graph4"("Y Input"=w355, "X Input"=w359) -> ("XY Graph"=→"R4":cluster{"X":dbl[], "Y":dbl[]}[])  [unwired: 8 in, 1 out]
              n225 = Index Array(array=w349, index=0) -> (element=w343:string)
              n226 = call "Convert to Dynamic Data6"("2D Array"=w363) -> ("Dynamic Data Type"=w362:dynamicdata)  [unwired: 3 in]
              n227 = call "Convert to Dynamic Data2"("2D Array"=w365) -> ("Dynamic Data Type"=w364:dynamicdata)  [unwired: 3 in]
              n228 = Index Array(array=w349, index=1) -> (element=w345:string)
              n229 = call "Build XY Graph2"("Y Input"=w364, "X Input"=w362) -> ("XY Graph"=→"T":cluster{"X":dbl[], "Y":dbl[]}[])  [unwired: 8 in, 1 out]
              n230 = property on="T" class="XYGraph (strict)"("Visible"=w376, "XScale.NameLbl.Text"=w337, "XScale.UnitLabel.Text"=w336) -> ()  [unwired: 2 in, 2 out]
              n231 = Index Array(array=w349, index=2) -> (element=w347:string)
              n232 = property on="T 2" class="XYGraph (strict)"("Active Plot"=0, "Plot.Plot Name"=w343, "XScale.NameLbl.Text"="Combo Box", "Visible"=w341) -> ()  [unwired: 2 in, 2 out]
              n233 = property on="T 3" class="XYGraph (strict)"("Active Plot"=0, "Plot.Plot Name"=w345, "XScale.NameLbl.Text"="Combo Box", "Visible"=w341) -> ()  [unwired: 2 in, 2 out]
              n234 = property on="R4" class="XYGraph (strict)"("Visible"=w341, "Plot.Plot Name"=w347, "XScale.NameLbl.Text"="Combo Box") -> ()  [unwired: 2 in, 2 out]
              "R [Ohm]" <- w374
            }
            frame #6 {
              n235 = Wait (ms)(milliseconds to wait="Reading Delay [ms]") -> ()  [unwired: 1 out]
            }
          }
          n236 = local read "Measure"() -> (w129:bool)
        }
      }
    }
  }
